vi "PH_SHS_Analysis_Calibrator.find latest calibration data file.vi"(4 "error in (no error)":errorcluster, 5 "Certain Camera Instance?":string, 6 "Wanted Method":enum16{"automatic", "manual"}(ring), 7 "get latest method depending":bool) -> (0 "error out":errorcluster, 1 "found something ...":bool, 2 "latest file":path)   [LabVIEW 2014, in "PH_SHS_Analysis_Calibrator.lvlib"]
doc: "This VI is made to find the latest SHS calibration data file at the hard disk. You can also select different parameters to preselect files."
uses:
  PH_SHS_Analysis_Calibrator.lvlib
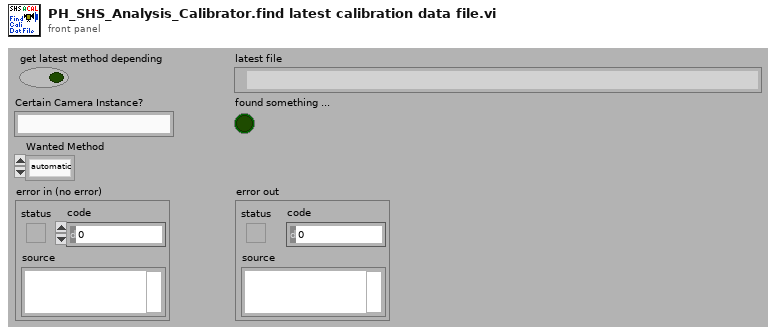
[diagram p1: front panel]
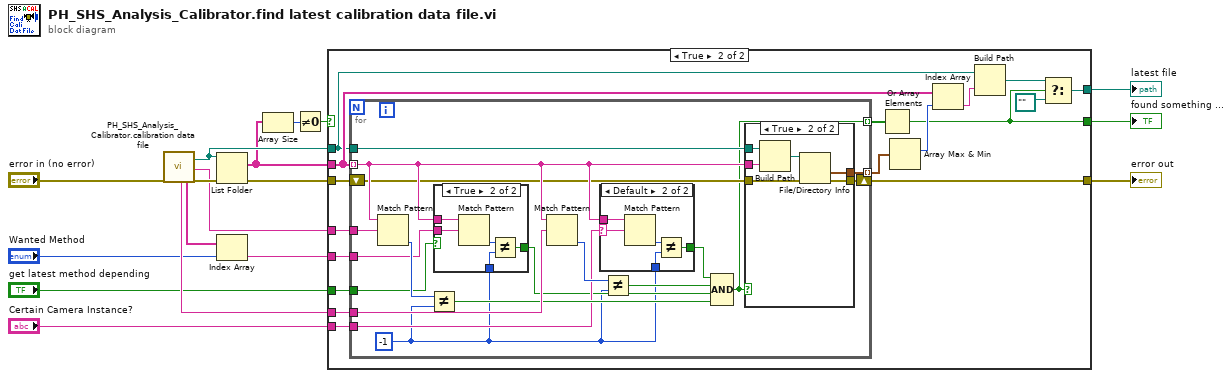
[diagram p0: block diagram]
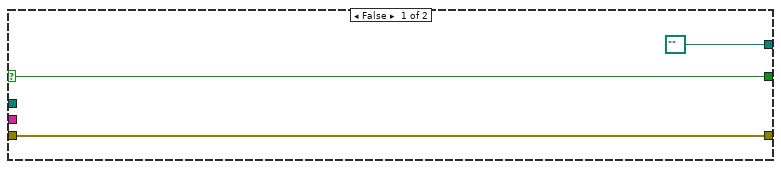
[diagram p2: hidden frame]
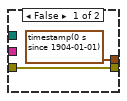
[diagram p3: hidden frame]
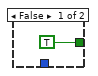
[diagram p4: hidden frame]
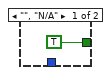
[diagram p5: hidden frame]
diagram:
  n1 = call "PH_SHS_Analysis_Calibrator.calibration data file.vi"("error in"="error in (no error)") -> ("File extension"=w14:string, "Methods"=w12:string[], "Directory path to save  SHS Analysis Calibration Data in"=w8:path, "Type of Data"=w15:string, "error out"=w16:errorcluster)  [unwired: 11 in, 3 out]
  n2 = List Folder(path=w8, error in=w16) -> (filenames=w5:string[], error out=w7:errorcluster)  [unwired: 2 in, 2 out]
  n3 = Index Array(array=w12, index="Wanted Method") -> (element=w9:string)
  n4 = Array Size(array=w5) -> (size(s)=w4:i32)
  n5 = Not Equal To 0?(x=w4) -> (x != 0?=w3:bool)
  n6 = case shown="True" w3 {
    selector: w3 -> [w20 _]
    tunnel: w15 -> [_ w37]
    tunnel: w14 -> [_ w36]
    tunnel: "Certain Camera Instance?" -> [_ w35]
    tunnel: "get latest method depending" -> [_ w34]
    tunnel: w9 -> [_ w33]
    tunnel: w8 -> [_ w25]
    tunnel: w7 -> [w19 w32]
    tunnel: [w19 w31] -> w6
    tunnel: w5 -> [_ w28]
    tunnel: [w20 w24] -> w2
    tunnel: [path "" ("appended path") w22] -> w1
    frame False {
    }
    frame True {
      n7 = for {
        tunnel: w28 -> [w43] mode=indexing
        tunnel: w37 -> [w55]
        tunnel: w36 -> [w54]
        tunnel: w35 -> [w48]
        tunnel: w34 -> [w47]
        tunnel: w33 -> [w45]
        tunnel: w25 -> [w42]
        shift-right: [w40] -> w31
        shift-left: w32 -> [w41]
        tunnel: [w39] -> w30 mode=indexing
        tunnel: [w38] -> w29 mode=indexing
        w44 = -1 ("y")
        n8 = Match Pattern(string=w43, regular expression=w55) -> (offset past match=w53:i32)  [unwired: 1 in, 3 out]
        n9 = Not Equal?(x=w53, y=w44) -> (x != y?=w50:bool)
        n10 = case shown="True" w47 {
          tunnel: w43 -> [_ w69]
          tunnel: [TRUE w67] -> w46
          tunnel: w44 -> [_ w66]
          tunnel: w45 -> [_ w65]
          frame False {
          }
          frame True {
            n11 = Match Pattern(string=w69, regular expression=w65) -> (offset past match=w68:i32)  [unwired: 1 in, 3 out]
            n12 = Not Equal?(x=w68, y=w66) -> (x != y?=w67:bool)
          }
        }
        n13 = Match Pattern(string=w43, regular expression=w54) -> (offset past match=w52:i32)  [unwired: 1 in, 3 out]
        n14 = case shown="Default" w48 {
          selector: w48 -> [_ w72]
          tunnel: w43 -> [_ w75]
          tunnel: [TRUE w73] -> w49
          tunnel: w44 -> [_ w71]
          frame "", "N/A" {
          }
          frame Default {
            n15 = Match Pattern(string=w75, regular expression=w72) -> (offset past match=w74:i32)  [unwired: 1 in, 3 out]
            n16 = Not Equal?(x=w74, y=w71) -> (x != y?=w73:bool)
          }
        }
        n17 = Not Equal?(x=w52, y=w44) -> (x != y?=w51:bool)
        n18 = Compound Arithmetic op=AND(w49, w51, w46, w50) -> (w38:bool)
        n19 = case shown="True" w38 {
          tunnel: w43 -> [_ w63]
          tunnel: w42 -> [_ w62]
          tunnel: w41 -> [w57 w60]
          tunnel: [w57 w59] -> w40
          tunnel: [timestamp(0 s since 1904-01-01) ("last mod") w58] -> w39
          frame False {
          }
          frame True {
            n20 = Build Path(base path=w62, name or relative path=w63) -> (appended path=w61:path)
            n21 = File/Directory Info(path=w61, error in=w60) -> (last mod=w58:timestamp, error out=w59:errorcluster)  [unwired: 5 out]
          }
        }
      }
      n22 = Or Array Elements(Boolean array=w29) -> (logical OR=w24:bool)
      n23 = Array Max & Min(array=w30) -> (max index (indices)=w27:i32)  [unwired: 3 out]
      n24 = Index Array(array=w28, index=w27) -> (element=w26:string)
      n25 = Build Path(base path=w25, name or relative path=w26) -> (appended path=w23:path)
      n26 = Select(t=w23, s=w24, f=path "") -> (s? t:f=w22:path)
    }
  }
  "latest file" <- w1
  "error out" <- w6
  "found something ..." <- w2
